vi "Launcher.vi"() -> ()   [LabVIEW 2023]
uses:
  Test Caller Actor/Test Caller Actor.lvclass
  Class Loader/Class Loader/Class Loader.lvclass
  <vilib>/ActorFramework/Stop Msg/Stop Msg.lvclass
  <vilib>/ActorFramework/Actor/Actor.lvclass
panel:
  in  "FQN (T)":bool=TRUE
  in  "Test Actor Number":i32=2
  in  "Stop Class Loader":bool
  out "error out":errorcluster
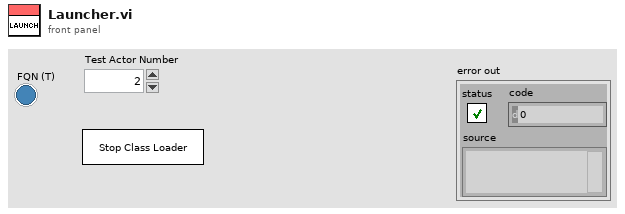
[diagram p1: front panel]
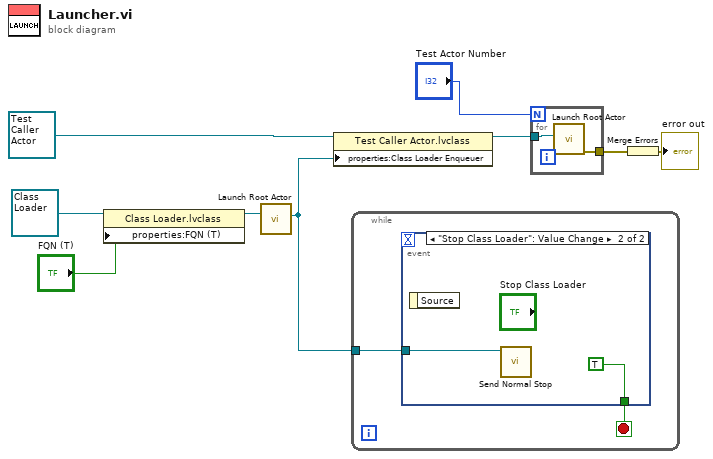
[diagram p0: block diagram]
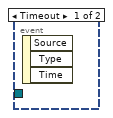
[diagram p2: hidden frame]
diagram:
  n1 = property class="Class Loader.lvclass"(reference=refnum<class "Class Loader.lvclass"> refnum ("Class Loader.lvlib:Class Loader.lvclass"), "properties:FQN (T)"="FQN (T)") -> (reference out=w2:refnum<class "Class Loader.lvclass">)  [unwired: 1 in, 1 out]
  n2 = call <vilib>:"Launch Root Actor.vi"("Actor"=w2) -> ("Actor's Enqueuer"=w4:refnum<class "Message Enqueuer.lvclass">)  [unwired: 9 in, 1 out]
  n3 = property class="Test Caller Actor.lvclass"(reference=refnum<class "Test Caller Actor.lvclass"> refnum ("Test Caller Actor.lvlib:Test Caller Actor.lvclass"), "properties:Class Loader Enqueuer"=w4) -> (reference out=w5:refnum<class "Test Caller Actor.lvclass">)  [unwired: 1 in, 1 out]
  n4 = while {
    tunnel: w4 -> [w11]
    stop <- w10 stop-if-true
    n5 = event shown="[1] \"Stop Class Loader\": Value Change" {
      selector: _ -> [_ _]
      dyn-events: _ -> [_ _]
      timeout: _ -> [_ _]
      tunnel: w11 -> [_ w13]
      tunnel: [_ TRUE] -> w10
      event Timeout {
        n6 = event-data() -> ()  [unwired: 1 in, 3 out]
      }
      event "Stop Class Loader": Value Change {
        n7 = event-data() -> ()  [unwired: 1 in, 1 out]
        n8 = call <vilib>:"Send Normal Stop.vi"("Message Enqueuer"=w13) -> ()  [unwired: 10 in, 1 out]
      }
    }
  }
  n9 = for {
    N: "Test Actor Number" -> [_]
    tunnel: [w15] -> w9
    tunnel: w5 -> [w14]
    n10 = call <vilib>:"Launch Root Actor.vi"("Actor"=w14) -> ("error out"=w15:errorcluster)  [unwired: 9 in, 1 out]
  }
  n11 = Merge Errors(w9) -> (→"error out":errorcluster)
